vi "2-4.vi"() -> ()   [LabVIEW 2014]
panel:
  out "응답프레임(일반 표기)":string
  in  "응답프레임(16진수 표기)":string
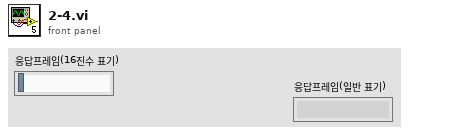
[diagram p1: front panel]
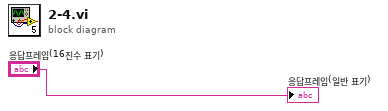
[diagram p0: block diagram]
diagram:
  "응답프레임(일반 표기)" <- "응답프레임(16진수 표기)"
